vi "Agilent DSO1000 Series Acquire Multiple Waveforms.vi"() -> ()   [LabVIEW 2020]
doc: "This example shows how to configure multiple channels and acquire waveforms from multiple channels."
uses:
  <instrlib>/Agilent DSO1000 Series/Public/Data/Read Waveform (Multiple).vi
  <vilib>/Utility/file.llb/Write Delimited Spreadsheet (DBL).vi
  <instrlib>/Agilent DSO1000 Series/Agilent DSO1000 Series.lvlib
panel:
  in  "Probe Attenuation (3: 1X)":u16(ring)=3 items=["0.001X", "0.01X", "0.1X", "1X", "10X", "100X", "1000X"]
  in  "Probe Attenuation (3: 1X)":u16(ring)=3 items=["0.001X", "0.01X", "0.1X", "1X", "10X", "100X", "1000X"]
  in  "Channel (1: Channel 1)":u16(ring)=2 items=["Channel 1"=1, "Channel 2"=2, "Channel 3"=3, "Channel 4"=4]
  in  "Channel (1: Channel 1)":u16(ring)=1 items=["Channel 1"=1, "Channel 2"=2, "Channel 3"=3, "Channel 4"=4]
  in  "Maximum Time (10000 ms)":u32=10000
  in  "Vertical Coupling (1: DC)":u16(ring)=1 items=["AC", "DC", "Ground"]
  in  "Vertical Coupling (1: DC)":u16(ring)=1 items=["AC", "DC", "Ground"]
  out "Waveform Data":waveform(dbl)[](graph)
  in  "VISA resource name":refnum<visa-resource-name>
  # "(c) 2009-2015 National Instruments.  ALL RIGHTS RESERVED."
  # "Channel A"
  # "Channel B"
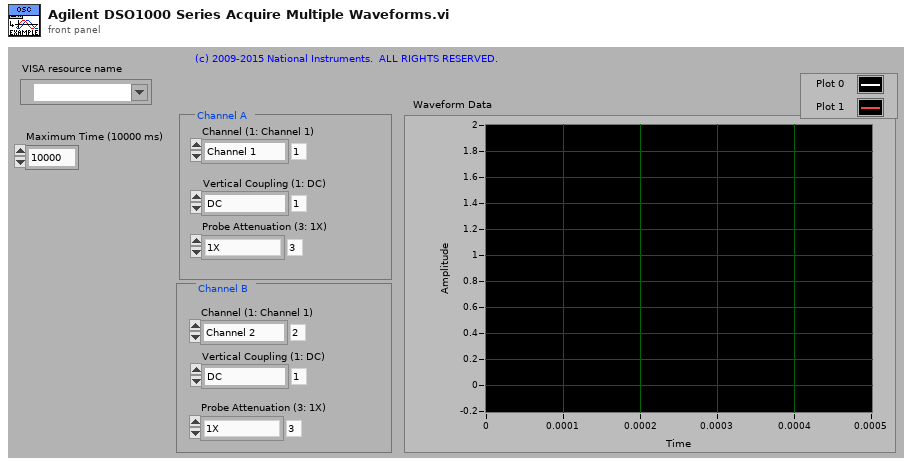
[diagram p1: front panel]
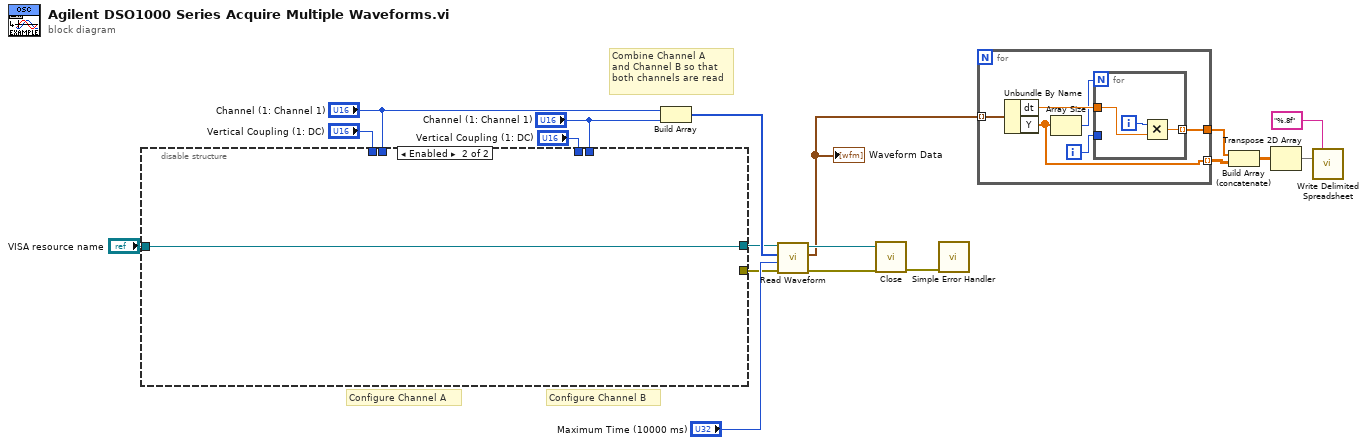
[diagram p0: block diagram]
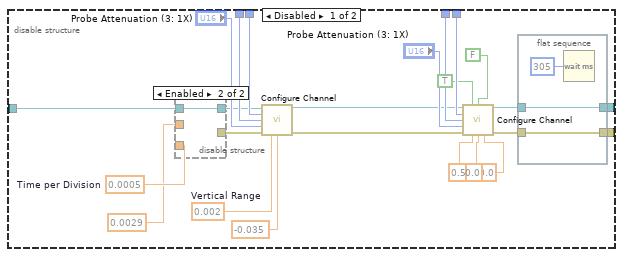
[diagram p2: hidden frame]
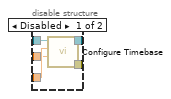
[diagram p3: hidden frame]
diagram:
  # "Combine Channel A\nand Channel B so that\nboth channels are read"
  # "Configure Channel B"
  # "Configure Channel A"
  n1 = disable-structure shown="Enabled" {
    disable-tunnel: "VISA resource name" -> [w42 w52]
    disable-tunnel: "Vertical Coupling (1: DC)" -> [w41 _]
    disable-tunnel: "Vertical Coupling (1: DC)" -> [w40 _]
    disable-tunnel: "Channel (1: Channel 1)" -> [w38 _]
    disable-tunnel: "Channel (1: Channel 1)" -> [w37 _]
    disable-tunnel: [w28 w52] -> w8
    disable-tunnel: [w26 _] -> w7
    frame Disabled {
      w39 = 0.0005  # Time per Division
      w32 = 0.002  # Vertical Range
      n2 = disable-structure shown="Enabled" {
        disable-tunnel: w39 -> [w47 _]
        disable-tunnel: w42 -> [w46 w48]
        disable-tunnel: [w45 w48] -> w31
        disable-tunnel: [w44 _] -> w30
        disable-tunnel: 0.0029 ("Time Delay (0.0 s)") -> [w43 _]
        frame Disabled {
          n3 = call <instrlib>:"Configure Timebase.vi"("Time Delay (0.0 s)"=w43, "Timebase (1E-6 s)"=w47, "VISA resource name"=w46) -> ("error out"=w44:errorcluster, "VISA resource name out"=w45:refnum<visa-resource-name>)  [unwired: 7 in]
        }
        frame Enabled {
        }
      }
      n4 = call <instrlib>:"Configure Channel.vi"("VISA resource name"=w31, "Channel (1: Channel 1)"=w38, "Vertical Coupling (1: DC)"=w41, "Probe Attenuation (3: 1X)"="Probe Attenuation (3: 1X)", "error in (no error)"=w30, "Vertical Range (10.0 V)"=w32, "Vertical Offset (0.0 V)"=-0.035) -> ("VISA resource name out"=w34:refnum<visa-resource-name>, "error out"=w33:errorcluster)  [unwired: 7 in]
      n5 = call <instrlib>:"Configure Channel.vi"("VISA resource name"=w34, "Enable Channel (T:Enable)"=TRUE, "Enable Invert  (F: Disable)"=FALSE, "Channel (1: Channel 1)"=w37, "Vertical Coupling (1: DC)"=w40, "Probe Attenuation (3: 1X)"="Probe Attenuation (3: 1X)", "error in (no error)"=w33, "Vertical Range (10.0 V)"=0.5, "Vertical Offset (0.0 V)"=0.0, "Max Input Frequency (0.0 Hz)"=0.0) -> ("VISA resource name out"=w29:refnum<visa-resource-name>, "error out"=w27:errorcluster)  [unwired: 4 in]
      n6 = flat-sequence {
        tunnel: w29 -> [w51]
        tunnel: [w51] -> w28
        tunnel: w27 -> [w50]
        tunnel: [w50] -> w26
        frame #0 {
          n7 = Wait (ms)(milliseconds to wait=u32 305) -> ()  [unwired: 1 out]
        }
      }
    }
    frame Enabled {
    }
  }
  n8 = Build Array("Channel (1: Channel 1)", "Channel (1: Channel 1)") -> (w11:u16[])
  n9 = call-poly <instrlib>:"Read Waveform.vi"("error in (no error)"=w7, "Maximum Time (10000 ms)"="Maximum Time (10000 ms)", "Channels"=w11, "VISA resource name"=w8) -> ("error out"=w13:errorcluster, "Waveform Data"=w6:waveform(dbl)[], "VISA resource name out"=w14:refnum<visa-resource-name>)  [unwired: 5 in]
  "Waveform Data" <- w6
  n10 = call <instrlib>:"Close.vi"("error in (no error)"=w13, "VISA resource name"=w14) -> ("error out"=w17:errorcluster)  [unwired: 9 in]
  n11 = call <vilib>:"Simple Error Handler.vi"("error in (no error)"=w17) -> ()  [unwired: 4 in, 5 out]
  n12 = for {
    tunnel: w6 -> [w56] mode=indexing
    tunnel: [w54] -> w5 mode=indexing
    tunnel: [w55] -> w4
    i -> [w57]
    n13 = Unbundle By Name(w56) -> ("dt"=w58:dbl, "Y"=w54:dbl[])
    n14 = Array Size(array=w54) -> (size(s)=w53:i32)
    n15 = for {
      N: w53 -> [_]
      tunnel: w57 -> [_]
      tunnel: w58 -> [w61]
      tunnel: [w60] -> w55 mode=indexing
      i -> [w59]
      n16 = Multiply(x=w59, y=w61) -> (x*y=w60:dbl)
    }
  }
  n17 = Build Array (concatenate)(w4, w5) -> (w3:dbl[][])
  n18 = Transpose 2D Array(2D array=w3) -> (transposed array=w2:dbl[][])
  n19 = call-poly <vilib>:"Write Delimited Spreadsheet.vi"("format (%.3f)"="%.8f", "2D data"=w2) -> ()  [unwired: 12 in, 2 out]
